vi "Is Instrument in Map.vi"(8 "error in":errorcluster, 10 "instrument type id":string, 11 "connection map in":refnum<class "Connection Map.lvclass">) -> (0 "error out":errorcluster, 2 "instrument in map":bool, 3 "connection map out":refnum<class "Connection Map.lvclass">)   [LabVIEW 2020, in "MeasurementLink Session Management.lvlib" / "Connection Map.lvclass"]
uses:
  Connection Map.lvclass
  Connection Map.lvclass/Connection Map.ctl
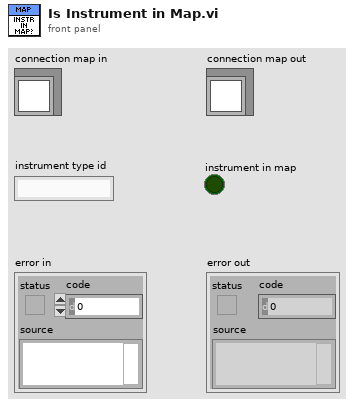
[diagram p1: front panel]
types:
  T1 = typedef "MeasurementLink Session Management.lvlib/Session Reservation.lvclass/Connection with Session.ctl" = cluster{"connection":T2, "session":variant}
  T2 = typedef "MeasurementLink Session Management.lvlib/Session Reservation.lvclass/Connection.ctl" = cluster{"pin or relay name":string, "site":i32, "instrument type id":string, "channel":string}
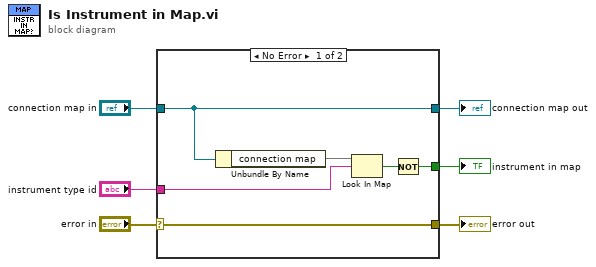
[diagram p0: block diagram]
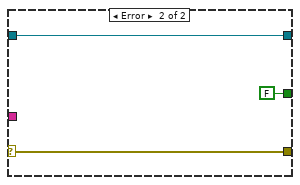
[diagram p2: hidden frame]
diagram:
  n1 = case shown="No Error" "error in" {
    selector: "error in" -> [w12 w15]
    tunnel: [w12 w15] -> w5
    tunnel: [w11 w14] -> w3
    tunnel: "connection map in" -> [w11 w14]
    tunnel: "instrument type id" -> [w9 _]
    tunnel: [w7 FALSE ("key not found?")] -> w1
    frame No Error {
      n2 = Unbundle By Name(w11) -> ("connection map"=w10:map{string, map{i32, map{string, T1}}})
      n3 = Look In Map(map=w10, key=w9) -> (key not found?=w8:bool)  [unwired: 1 in, 1 out]
      n4 = Not(x=w8) -> (.not. x?=w7:bool)
    }
    frame Error {
    }
  }
  "error out" <- w5
  "connection map out" <- w3
  "instrument in map" <- w1
